vi "Untitled 8 (SubVI).vi"(8 "error in (no error)":errorcluster, 11 ".NET Refnum in":refnum<k24>) -> (0 "error out":errorcluster, 3 "Checkbox":bool)   [LabVIEW 2021, in "Open Xml.lvlib"]
uses:
  Open Xml.lvlib
  D:/git/Open-Xml-LabVIEW/dll/DocumentFormat.OpenXml.dll
  dll/DocumentFormat.OpenXml.dll
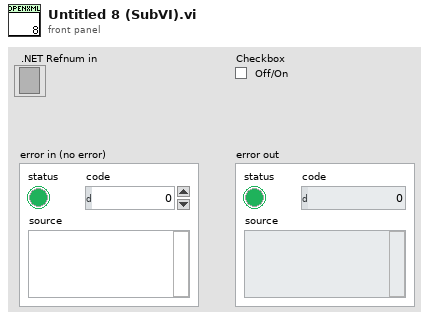
[diagram p1: front panel]
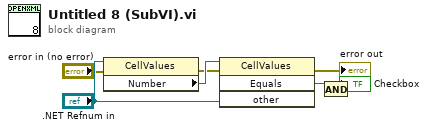
[diagram p0: block diagram]
diagram:
  n1 = property class="CellValues"(reference=".NET Refnum in", error in="error in (no error)") -> (error out=w2:errorcluster, "Number"=w5:refnum<k24>)  [unwired: 1 out]
  n2 = invoke class="CellValues" method="Equals"(reference=w5, error in=w2, "other"=".NET Refnum in") -> (error out=→"error out":errorcluster, "Equals"=w4:bool)  [unwired: 1 in, 2 out]
  n3 = And(x=w4) -> (x .and. y?=→"Checkbox":bool)  [unwired: 1 in]
